vi "IMAQdx_FindCamAttributes.vi"() -> ()   [LabVIEW 2018]
uses:
  <vilib>/userdefined/High Color/IMAQdx.ctl
  <vilib>/vision/driver/IMAQdx.llb/IMAQdx Attribute Type.ctl
  <vilib>/vision/driver/NI_Vision_Acquisition_Software.lvlib
  <resource>/objmgr/imaqdx.rc
panel:
  in  "下拉列表":u16(ring) items=["Freerun"=0, "Line1"=1, "Line2"=2, "FixedRate"=5, "Software"=6]
  out "ValueBool":bool
  out "DisplayName 2":string
  out "EnumValues[]":u32[](array[numeric])
  out "EnumStrings[]":string[](array[string])
  out "Units":string
  out "MinDBL":dbl
  out "MaxDBL":dbl
  out "ValueDBL":dbl
  out "DisplayName":string
  out "Description":string
  out "元素索引":i32
  out "Attribute Name":string
  out "Attribute Information Array":T2(array[cluster])
  in  "Camera Name In":T3 caption="Session In"
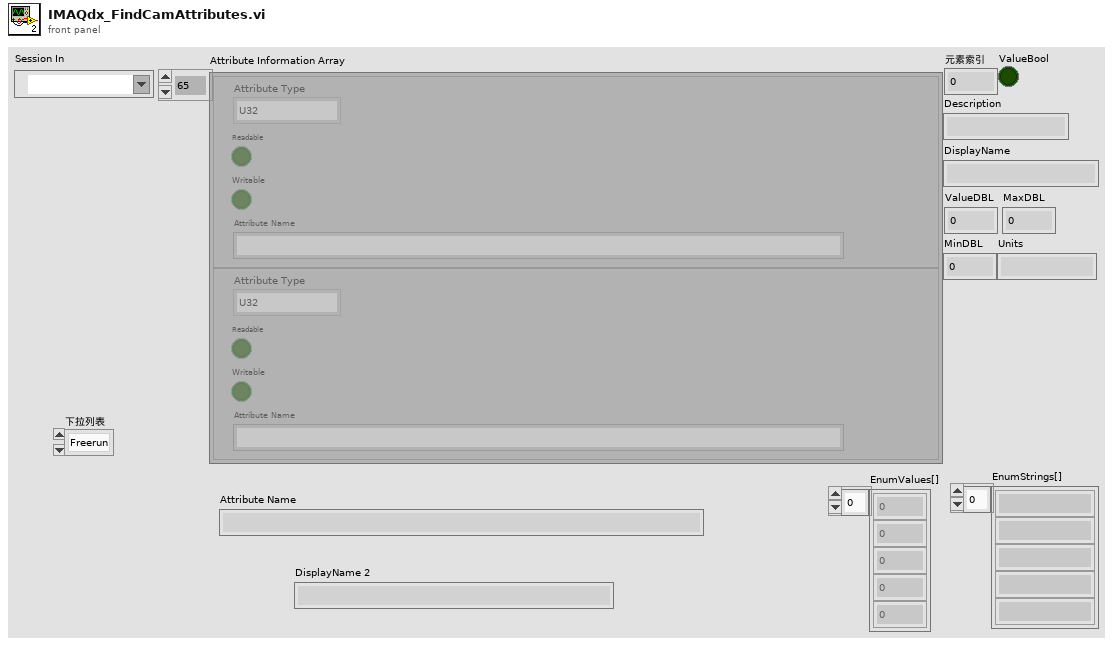
[diagram p1: front panel]
types:
  T1 = typedef "NI_Vision_Acquisition_Software.lvlib/IMAQdx Attribute Type.ctl" = enum32{"U32", "I64", "DBL", "String", "Enum", "Bool", "Command"}
  T2 = cluster{"Attribute Type":T1, "Readable":bool, "Writable":bool, "Attribute Name":string}[]
  T3 = typedef "IMAQdx.ctl" = refnum<k21>
  T4 = cluster{"Attribute Type":T1, "Readable":bool, "Writable":bool, "Attribute Name":string}
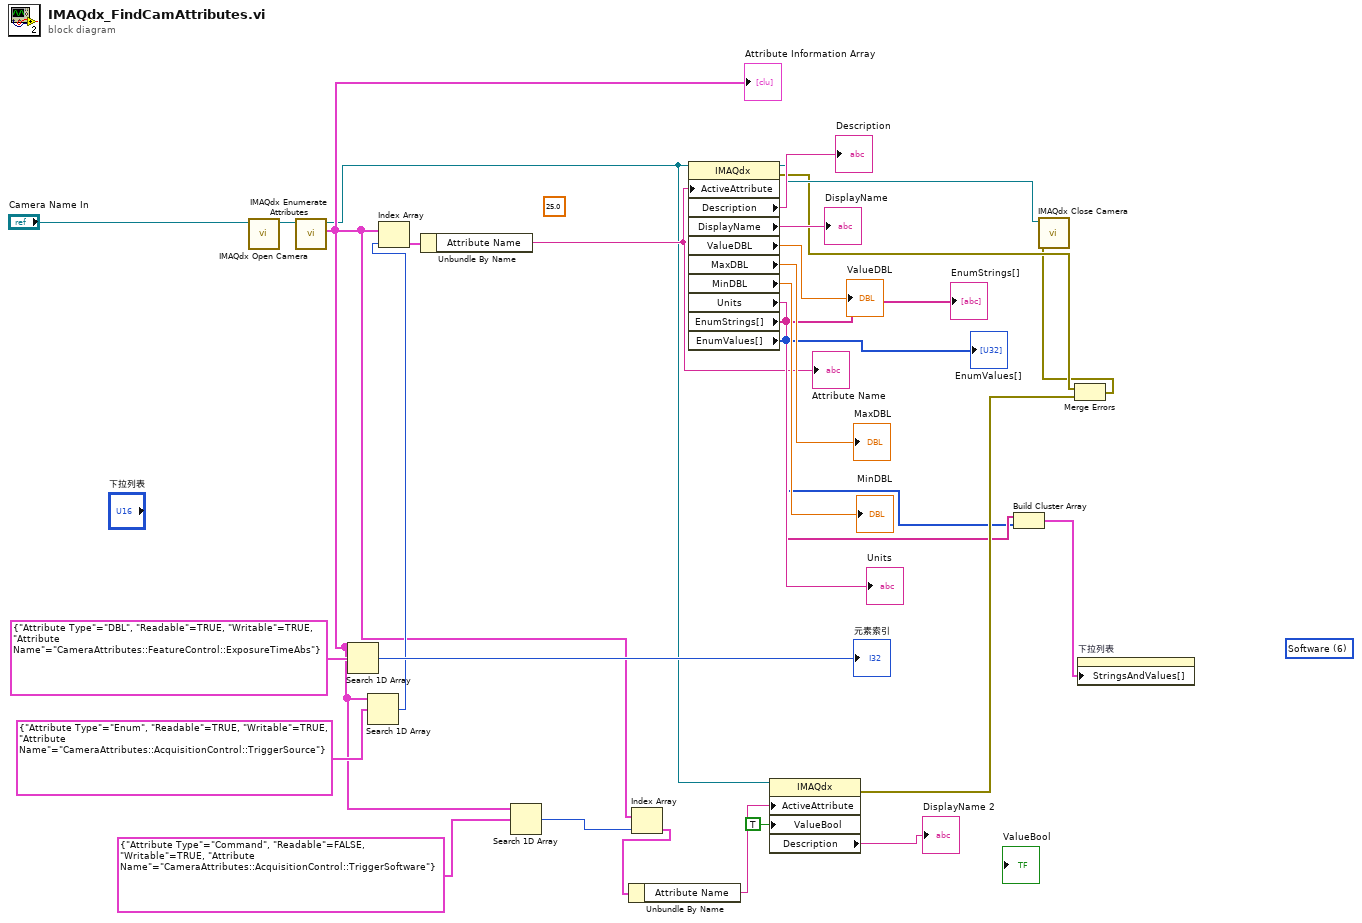
[diagram p0: block diagram]
diagram:
  (unwired) u16 6 items=["Freerun"=0, "Line1"=1, "Line2"=2, "FixedRate"=5, "Software"=6] ("下拉列表 2")
  (unwired) 25.0 ("ValueDBL")
  n1 = call <vilib>:"IMAQdx Open Camera.vi"("Session In"="Camera Name In") -> ("Session Out"=w28:T3)  [unwired: 9 in, 1 out]
  n2 = call <vilib>:"IMAQdx Enumerate Attributes.vi"("Session In"=w28) -> ("Attribute Information Array"=w15:T2, "Session Out"=w9:T3)  [unwired: 3 in, 6 out]
  "Attribute Information Array" <- w15
  n3 = Search 1D Array(1D array=w15, element=T4 {"Attribute Type"=enum."DBL", "Readable"=TRUE, "Writable"=TRUE, "Attribute Name"="CameraAttributes::FeatureControl::ExposureTimeAbs"} ("元素")) -> (index of element=→"元素索引":i32)  [unwired: 1 in]
  n4 = Search 1D Array(1D array=w15, element=T4 {"Attribute Type"=enum."Enum", "Readable"=TRUE, "Writable"=TRUE, "Attribute Name"="CameraAttributes::AcquisitionControl::TriggerSource"} ("元素")) -> (index of element=w16:i32)  [unwired: 1 in]
  n5 = Index Array(array=w15, index=w16) -> (element=w26:T4)
  n6 = Unbundle By Name(w26) -> ("Attribute Name"=w13:string)
  "Attribute Name" <- w13
  n7 = Search 1D Array(1D array=w15, element=T4 {"Attribute Type"=enum."Command", "Readable"=FALSE, "Writable"=TRUE, "Attribute Name"="CameraAttributes::AcquisitionControl::TriggerSoftware"} ("元素")) -> (index of element=w14:i32)  [unwired: 1 in]
  n8 = Index Array(array=w15, index=w14) -> (element=w12:T4)
  n9 = Unbundle By Name(w12) -> ("Attribute Name"=w11:string)
  n10 = property class="IMAQdx"(reference=w9, "ActiveAttribute"=w13) -> (reference out=w8:T3, error out=w7:errorcluster, "Description"=→"Description":string, "DisplayName"=→"DisplayName":string, "ValueDBL"=→"ValueDBL":dbl, "MaxDBL"=→"MaxDBL":dbl, "MinDBL"=→"MinDBL":dbl, "Units"=→"Units":string, "EnumStrings[]"=w3:string[], "EnumValues[]"=w2:u32[])  [unwired: 1 in]
  "EnumStrings[]" <- w3
  "EnumValues[]" <- w2
  n11 = property class="IMAQdx"(reference=w9, "ActiveAttribute"=w11, "ValueBool"=TRUE) -> (error out=w6:errorcluster, "Description"=→"DisplayName 2":string)  [unwired: 1 in, 1 out]
  n12 = Build Cluster Array(w3, w2) -> (w1:cluster{string, u32}[])
  n13 = Merge Errors(w7, w6) -> (w5:errorcluster)
  n14 = call <vilib>:"IMAQdx Close Camera.vi"("error in"=w5, "Session In"=w8) -> ()  [unwired: 9 in, 1 out]
  n15 = property on="下拉列表" class="Ring (严格)"("StringsAndValues[]"=w1) -> ()  [unwired: 2 in, 2 out]
